vi "Caraya Verify Hello Caraya.vi"   [LabVIEW 2020]
uses:
  Caraya.Extension/Caraya.Extension.lvlib
  <vilib>/addons/_JKI Toolkits/Caraya/classes/Test/Test.lvclass
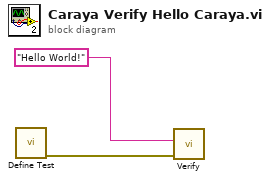
[diagram p0: block diagram]
diagram:
  n1 = call <vilib>:"Define Test.vi"() -> ("error out"=w1:errorcluster)  [unwired: 10 in, 1 out]
  n2 = call "Verify.vi"("error in"=w1, "Test Data"="Hello World!") -> ()  [unwired: 9 in, 1 out]
